vi "Filter relevant controls.vi"(11 "Rules":T1[](array[typedef])) -> (2 "Relevant Rules":T1[][](array[typedef]), 3 "Relevent Controls":string[](array[string]))   [LabVIEW 2019, in "LSS.lvlib"]
doc: "Filter out any rules that may not be relevent"
uses:
  LSS.lvlib
  Controls/Rule.ctl
  Controls/Criteria.ctl
  Controls/Comparison Types.ctl
  Controls/Effects.ctl
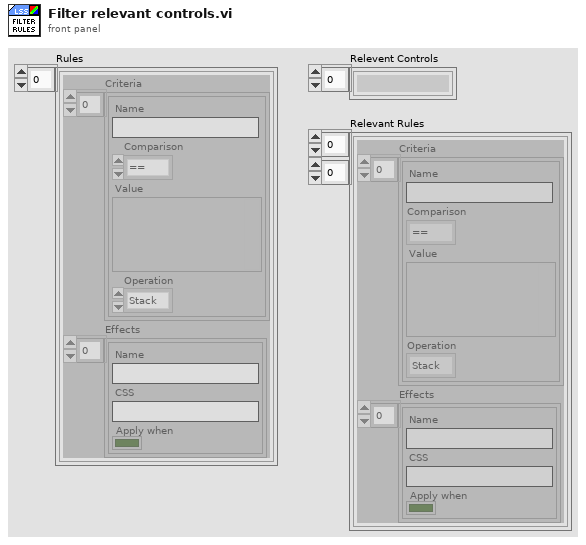
[diagram p1: front panel]
types:
  T1 = typedef "LSS.lvlib/Rule.ctl" = cluster{"Criteria":T2[], "Effects":T4[]}
  T2 = typedef "LSS.lvlib/Criteria.ctl" = cluster{"Name":string, "Comparison":T3, "Value":variant, "Operation":enum16{"Stack", "&&", "||"}}
  T3 = typedef "LSS.lvlib/Comparison Types.ctl" = enum16{"==", "!=", "<", ">", "<=", ">="}
  T4 = typedef "LSS.lvlib/Effects.ctl" = cluster{"Name":string, "CSS":string, "Apply when":bool}
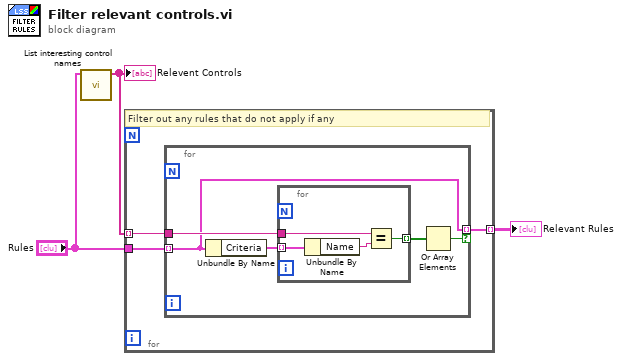
[diagram p0: block diagram]
diagram:
  n1 = call "List interesting control names.vi"("Rules"="Rules") -> ("Relevant Controls"=w1:string[])  [unwired: 9 in, 1 out]
  "Relevent Controls" <- w1
  n2 = for {
    tunnel: w1 -> [w5] mode=indexing
    tunnel: "Rules" -> [w6]
    tunnel: [w4] -> w3 mode=indexing
    # "Filter out any rules that do not apply if any"
    n3 = for {
      tunnel: w6 -> [w8] mode=indexing
      tunnel: w5 -> [w10]
      tunnel: [w8] -> w4 mode=indexing if=w7
      n4 = Unbundle By Name(w8) -> ("Criteria"=w11:T2[])
      n5 = for {
        tunnel: w11 -> [w15] mode=indexing
        tunnel: w10 -> [w13]
        tunnel: [w12] -> w9 mode=indexing
        n6 = Unbundle By Name(w15) -> ("Name"=w14:string)
        n7 = Equal?(x=w13, y=w14) -> (x = y?=w12:bool)
      }
      n8 = Or Array Elements(Boolean array=w9) -> (logical OR=w7:bool)
    }
  }
  "Relevant Rules" <- w3
